vi "globalSetUp.vi"(8 "error in (no error)":errorcluster, 11 "testcase-CSMNonCSMCallerSupportAPI.lvclass in":refnum<class "testcase-CSMNonCSMCallerSupportAPI.lvclass">) -> (0 "error out":errorcluster, 3 "testcase-CSMNonCSMCallerSupportAPI.lvclass out":refnum<class "testcase-CSMNonCSMCallerSupportAPI.lvclass">)   [LabVIEW 2017, in "testcase-CSMNonCSMCallerSupportAPI.lvclass"]
uses:
  testcase-CSMNonCSMCallerSupportAPI.lvclass
  <vilib>/addons/_JKI Toolkits/VI Tester/TestCase.llb/TestCase.lvclass
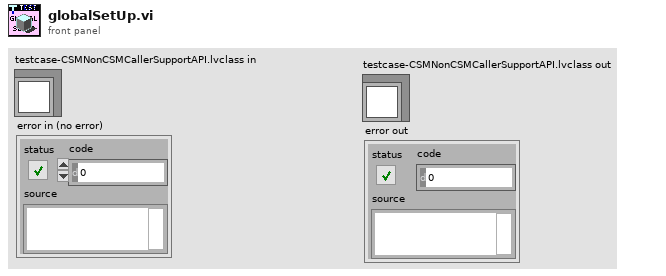
[diagram p1: front panel]
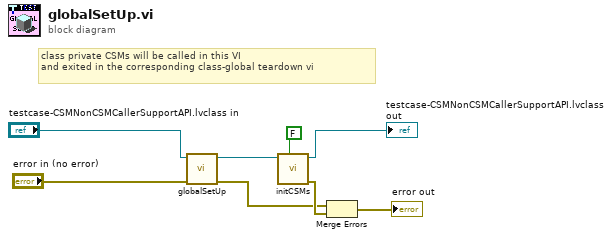
[diagram p0: block diagram]
diagram:
  # "class private CSMs will be called in this VI\nand exited in the corresponding class-global teardown vi"
  n1 = call-parent "globalSetUp.vi"("error in (no error)"="error in (no error)", "TestCase in"="testcase-CSMNonCSMCallerSupportAPI.lvclass in") -> ("error out"=w2:errorcluster, "TestCase out"=w5:refnum<class "testcase-CSMNonCSMCallerSupportAPI.lvclass">)  [unwired: 8 in]
  n2 = call "initCSMs.vi"("Enable building lvlibp?"=FALSE, "TestCase in"=w5) -> ("error out"=w6:errorcluster, "TestCase out"=→"testcase-CSMNonCSMCallerSupportAPI.lvclass out":refnum<class "testcase-CSMNonCSMCallerSupportAPI.lvclass">)  [unwired: 8 in]
  n3 = Merge Errors(w2, w6) -> (→"error out":errorcluster)
